vi "Read Parameters Value.vi"(8 "error in (no error)":errorcluster, 11 "Mag Lab Root in":refnum<class "Mag Lab Root.lvclass">) -> (0 "error out":errorcluster, 2 "Parameters Value":variant, 3 "Mag Lab Root out":refnum<class "Mag Lab Root.lvclass">)   [LabVIEW 2015, in "Mag Lab Root.lvclass"]
uses:
  Mag Lab Root.lvclass
  Mag Lab Properties/Mag Lab Parameters.lvclass
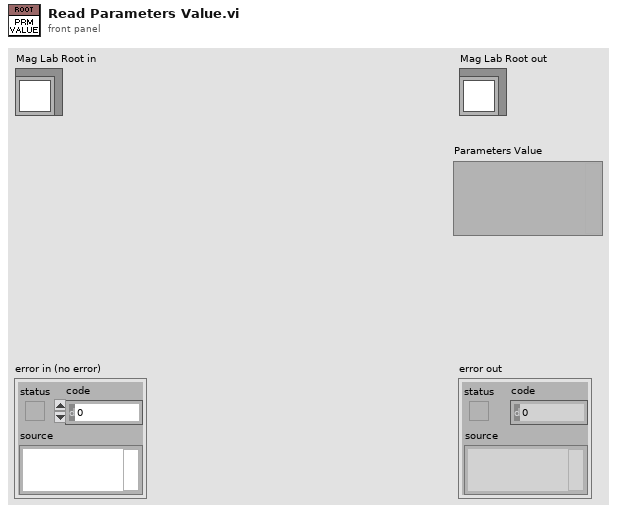
[diagram p1: front panel]
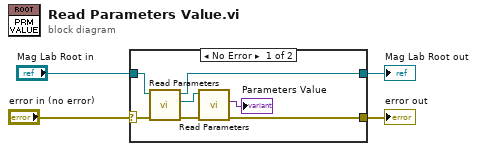
[diagram p0: block diagram]
diagram:
  n1 = case shown="No Error" "error in (no error)" {
    selector: "error in (no error)" -> [w8 w13]
    tunnel: [w5 w13] -> w3
    tunnel: [w10 w12] -> w1
    tunnel: "Mag Lab Root in" -> [w11 w12]
    frame No Error {
      n2 = call-dynamic "Read Parameters.vi"("error in (no error)"=w8, "Mag Lab Root in"=w11) -> ("error out"=w6:errorcluster, "Mag Lab Parameters.lvclass"=w9:refnum<class "Mag Lab Parameters.lvclass">, "Mag Lab Root out"=w10:refnum<class "Mag Lab Root.lvclass">)  [unwired: 7 in]
      n3 = call-dynamic "Read Parameters.vi"("error in (no error)"=w6, "Mag Lab Parameters in"=w9) -> ("error out"=w5:errorcluster, "Parameters"=→"Parameters Value":variant)  [unwired: 7 in, 1 out]
    }
    frame Error {
    }
  }
  "error out" <- w3
  "Mag Lab Root out" <- w1
